vi "Actuator Transaction Lists.vi"(0 "Source":T1, 2 "error in (no error)":errorcluster) -> (3 "Actuator Data":T2[](array[typedef]), 4 "Actuator Volts":T2[](array[typedef]), 6 "error out":errorcluster)   [LabVIEW 2009]
uses:
  Dataset Transaction Id.ctl
  Dataset Source.ctl
  Dataset Type.ctl
  Apps/Yes No Button.ctl
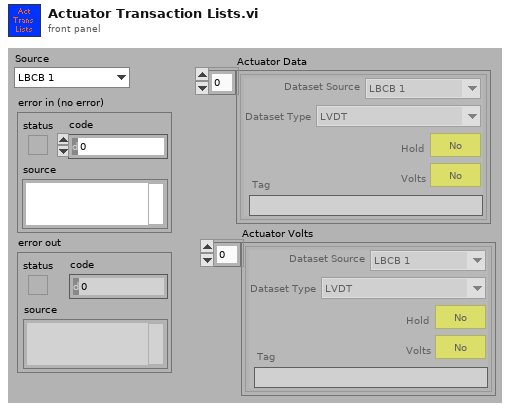
[diagram p1: front panel]
types:
  T1 = typedef "Dataset Source.ctl" = enum16{"LBCB 1", "LBCB 2", "Combined", "External Sensors"}
  T2 = typedef "Dataset Transaction Id.ctl" = cluster{"Dataset Source":T1, "Dataset Type":T3, "Hold":T4, "Volts":T4, "Tag":string}
  T3 = typedef "Dataset Type.ctl" = enum16{"LVDT", "Load Cell", "Actuator Command", "Servo Error", "Displacement Command", "Displacement", "Force"}
  T4 = typedef "Yes No Button.ctl" = bool
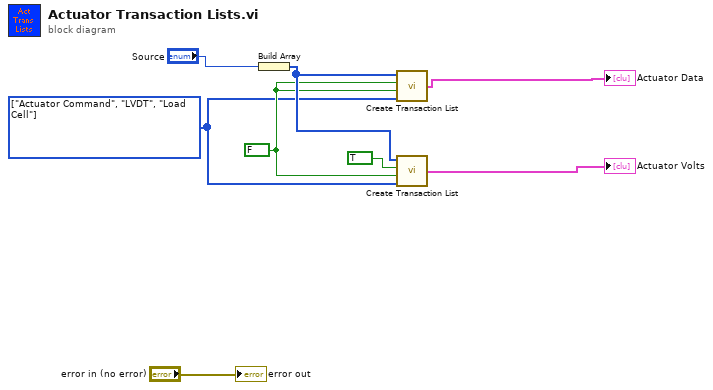
[diagram p0: block diagram]
diagram:
  w2 = T3[] [enum."Actuator Command", enum."LVDT", enum."Load Cell"] items=["LVDT", "Load Cell", "Actuator Command", "Servo Error", "Displacement Command", "Displacement", "Force"] ("Types")
  w4 = FALSE ("Volts")
  n1 = Build Array("Source") -> (w5:T1[])
  n2 = call "Create Transaction List.vi"("Types"=w2, "Hold"=w4, "Volts"=w4, "Sources"=w5) -> ("Transactions"=→"Actuator Data":T2[])
  n3 = call "Create Transaction List.vi"("Types"=w2, "Hold"=w4, "Volts"=TRUE, "Sources"=w5) -> ("Transactions"=→"Actuator Volts":T2[])
  "error out" <- "error in (no error)"
